vi "gps_speed_estimation.vi"(0 "LatitudePrev":dbl, 1 "LongitudePrev":dbl, 2 "Latitude":dbl, 3 "Speed Threshold":dbl, 4 "Longitude":dbl) -> (5 "GPS":T1, 6 "Arm System":bool)   [LabVIEW 2023]
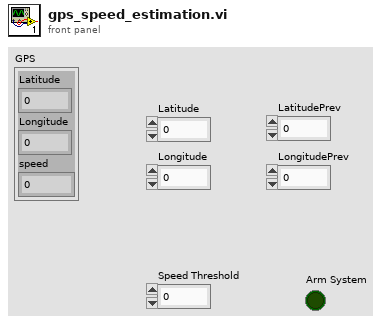
[diagram p1: front panel]
types:
  T1 = cluster{"Latitude":dbl, "Longitude":dbl, "speed":dbl}
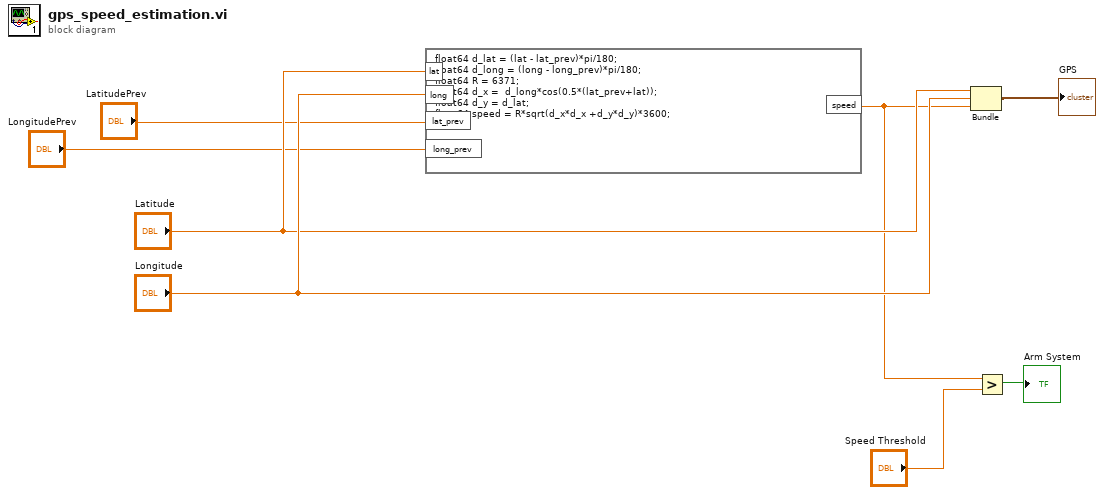
[diagram p0: block diagram]
diagram:
  n1 = formula code="float64 d_lat = (lat - lat_prev)*pi/180;\nfloat64 d_long = (long - long_prev)*pi/180;\nfloat64 R = 6371;\nfloat64 d_x =  d_long*cos(0.5*(lat_prev+lat));\nfloat64 d_y = d_lat;\nfloat64 speed = R*sqrt(d_x*d_x +d_y*d_y)*3600;"("lat"="Latitude", "lat_prev"="LatitudePrev", "long"="Longitude", "long_prev"="LongitudePrev") -> ("speed"=w3:dbl)
  n2 = Bundle("Latitude"="Latitude", "Longitude"="Longitude", w3) -> (→"GPS":cluster{"Latitude":dbl, "Longitude":dbl, dbl})  [unwired: 1 in]
  n3 = Greater?(x=w3, y="Speed Threshold") -> (0:→"Arm System":bool)
